vi "TDMS Filter Properties.vi"(5 "Property Values":variant[](array[variant]), 7 "Property Names":string[](array[string])) -> (4 "Filtered Property Values":variant[](array[variant]), 6 "Filtered Property Names":string[](array[string]))   [LabVIEW 2020, in "Utilities.lvlib"]
doc: "Removes internal TDMS properties from the name and value pairs given."
uses:
  Utilities.lvlib
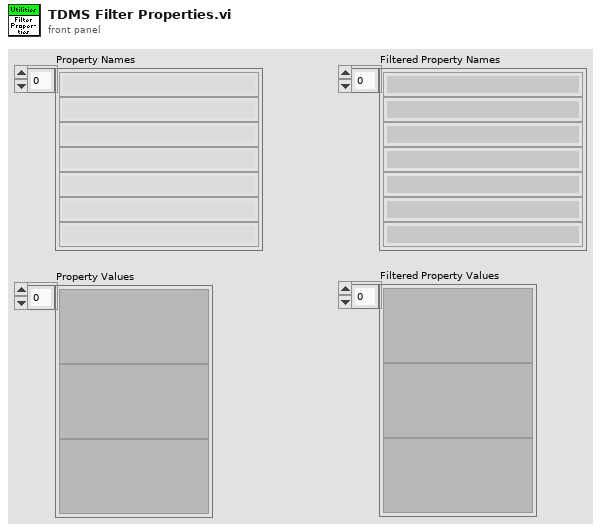
[diagram p1: front panel]
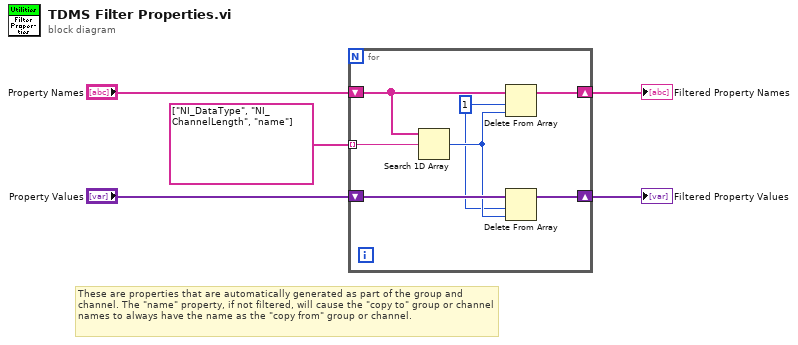
[diagram p0: block diagram]
diagram:
  # "These are properties that are automatically generated as part of the group and channel. The \"name\" property, if not filtered, will cause the \"copy to\" group or channel names to always have the name as the \"copy from\" group or channel."
  n1 = for {
    tunnel: string[] ["NI_DataType", "NI_ChannelLength", "name"] -> [w12] mode=indexing
    shift-right: [w9] -> w2
    shift-left: "Property Values" -> [w10]
    shift-right: [w8] -> w1
    shift-left: "Property Names" -> [w11]
    w6 = 1 ("length")
    n2 = Search 1D Array(1D array=w11, element=w12) -> (index of element=w7:i32)  [unwired: 1 in]
    n3 = Delete From Array(array=w11, length=w6, index=w7) -> (array with subset deleted=w8:string[])  [unwired: 1 out]
    n4 = Delete From Array(array=w10, length=w6, index=w7) -> (array with subset deleted=w9:variant[])  [unwired: 1 out]
  }
  "Filtered Property Names" <- w1
  "Filtered Property Values" <- w2
